vi "FromRepo.vi"(8 "error in":errorcluster, 9 "from repo cluster":T2, 10 "repository in":refnum<class "NISE_CEF_Repository.lvclass">, 11 "module editor node in":refnum<class "module editor node.lvclass">) -> (0 "error out":errorcluster, 2 "repository out":refnum<class "NISE_CEF_Repository.lvclass">, 3 "module editor node out":T1)   [LabVIEW 2013, in "PL Framework Configuration Tool.lvlib" / "module editor node.lvclass"]
doc: "Grabs information from the Repo and stores it in the nodes."
uses:
  module editor node.lvclass
  <vilib>/CEF_TreeControl/Repository/NISE_CEF_Repository.lvclass
  <vilib>/CEF_TreeControl/Node/FromRepoCluster.ctl
  <vilib>/CEF_TreeControl/Node/NodeRef.ctl
  <vilib>/CEF_TreeControl/Node/NISE_CEF_Node.lvclass
  <vilib>/NI/Tag Bus Module Framework/module configuration/TBM module configuration.lvclass
  Framework Configuration Classes/platypus configuration/engines cluster.ctl
  <vilib>/NI/Module Execution Interface/Engine Configuration/engine configuration.lvclass
  Framework Configuration Classes/platypus configuration/PLConfigurationSerializer.lvlib
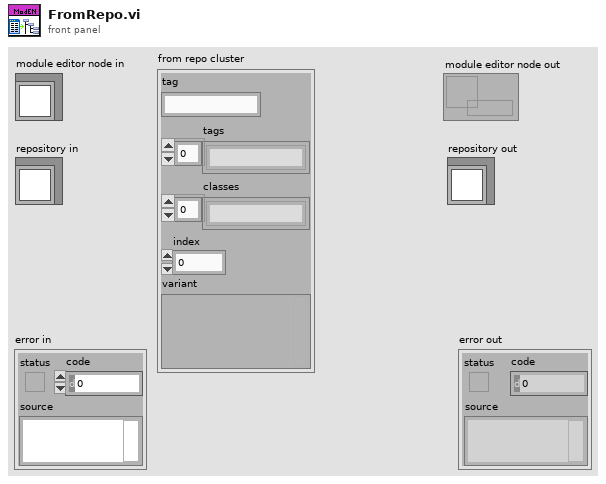
[diagram p1: front panel]
types:
  T1 = typedef "NISE_CEF_Node.lvclass/NodeRef.ctl" = refnum<data-value>
  T2 = typedef "NISE_CEF_Node.lvclass/FromRepoCluster.ctl" = cluster{"tag":string, "tags":string[], "classes":string[], "index":i32, "variant":variant}
  T3 = typedef "PLConfigurationSerializer.lvlib/engines cluster.ctl" = cluster{"engine configuration":refnum<class "engine configuration.lvclass">, "modules":refnum<class "TBM module configuration.lvclass">[]}
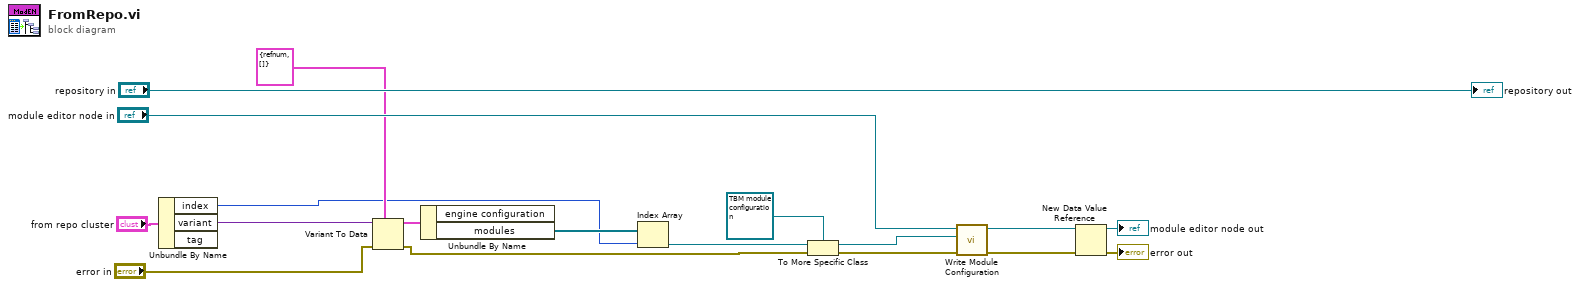
[diagram p0: block diagram]
diagram:
  n1 = Unbundle By Name("from repo cluster") -> ("index"=w3:i32, "variant"=w16:variant)  [unwired: 1 out]
  n2 = Variant To Data(error in="error in", type=T3 {"engine configuration"=refnum, "modules"=[]} ("engines cluster"), Variant=w16) -> (data=w15:T3, error out=w6:errorcluster)
  n3 = Unbundle By Name(w15) -> ("modules"=w14:refnum<class "TBM module configuration.lvclass">[])  [unwired: 1 out]
  n4 = Index Array(array=w14, index=w3) -> (element=w8:refnum<class "TBM module configuration.lvclass">)
  n5 = To More Specific Class(target class=refnum<class "TBM module configuration.lvclass"> refnum ("component configuration.lvclass"), reference=w8, error in=w6) -> (specific class reference=w1:refnum<class "TBM module configuration.lvclass">, error out=w2:errorcluster)
  n6 = call "Write Module Configuration.vi"("error in"=w2, "module configuration"=w1, "Module Editor Node in"="module editor node in") -> ("error out"=w10:errorcluster, "Module Editor Node out"=w12:refnum<class "module editor node.lvclass">)  [unwired: 7 in]
  n7 = New Data Value Reference(data value=w12, error in=w10) -> (data value reference=→"module editor node out":refnum<data-value>, error out=→"error out":errorcluster)
  "repository out" <- "repository in"
